vi "Update New Plugin by Reference.vi"(8 "error in (no error)":errorcluster, 10 "Plugin Types Tree":refnum<vi>, 11 "New Plugin Control":refnum<vi>) -> (0 "error out":errorcluster)   [LabVIEW 2021, in "CIF_Manager_UI.lvclass"]
uses:
  CIF_Manager_UI.lvclass
  Typedef/New Plugin.ctl
  CIF_Manager_UI.lvclass/CIF_Manager_UI.ctl
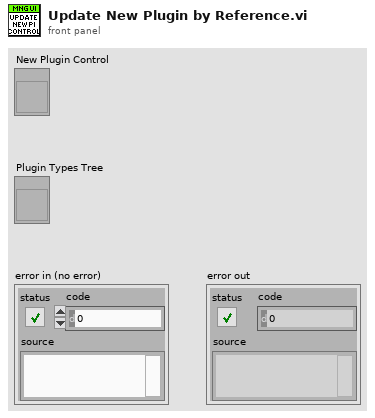
[diagram p1: front panel]
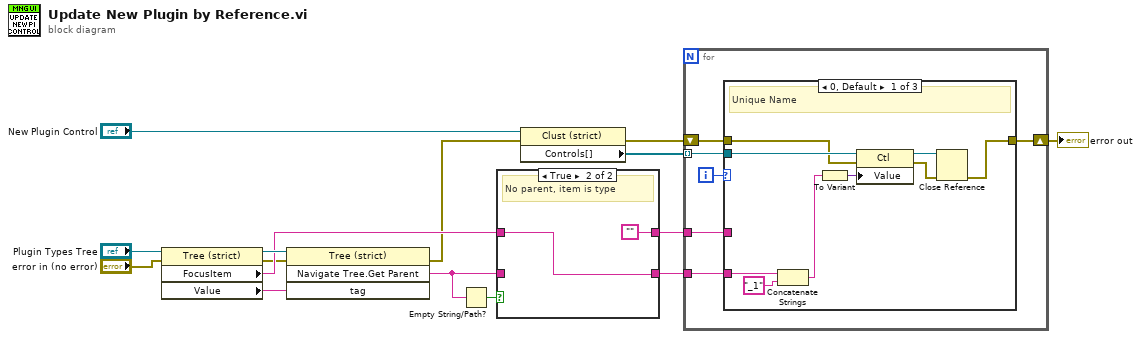
[diagram p0: block diagram]
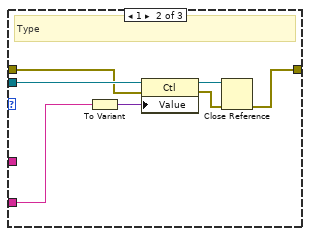
[diagram p3: hidden frame]
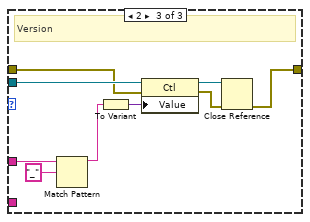
[diagram p4: hidden frame]
diagram:
  n1 = property class="Tree (strict)"(reference="Plugin Types Tree", error in="error in (no error)") -> (error out=w7:errorcluster, "FocusItem"=w8:string, "Value"=w13:string)  [unwired: 1 out]
  n2 = invoke class="Tree (strict)" method="Navigate Tree.Get Parent"(reference="Plugin Types Tree", error in=w7, "tag"=w13) -> (error out=w6:errorcluster, "Navigate Tree:Get Parent"=w9:string)  [unwired: 1 in, 2 out]
  n3 = Empty String/Path?(string/path=w9) -> (empty?=w10:bool)
  n4 = case shown="True" w10 {
    tunnel: w9 -> [w15 _]
    tunnel: w8 -> [w16 w18]
    tunnel: [w16 ""] -> w4
    tunnel: [w15 w18] -> w5
    frame False {
      # "Parent is type, item is version"
    }
    frame True {
      # "No parent, item is type"
    }
  }
  n5 = property class="Clust (strict)"(reference="New Plugin Control", error in=w6) -> (error out=w3:errorcluster, "Controls[]"=w14:refnum<vi>[])  [unwired: 1 out]
  n6 = for {
    tunnel: w14 -> [w23] mode=indexing
    tunnel: w5 -> [w22]
    tunnel: w4 -> [w21]
    shift-right: [w19] -> w1
    shift-left: w3 -> [w20]
    i -> [w24]
    n7 = case shown="0, Default" w24 {
      tunnel: w23 -> [w32 w40 w49]
      tunnel: w22 -> [w28 w38 _]
      tunnel: w21 -> [_ _ w43]
      tunnel: w20 -> [w30 w37 w47]
      tunnel: [w33 w34 w44] -> w19
      frame 0, Default {
        # "Unique Name"
        n8 = Concatenate Strings(w28, "_1" ("string")) -> (w26:string)
        n9 = To Variant(anything=w26) -> (Variant=w25:variant)
        n10 = property class="Ctl"(reference=w32, error in=w30, "Value"=w25) -> (reference out=w31:refnum<vi>, error out=w29:errorcluster)
        n11 = Close Reference(reference=w31, error in (no error)=w29) -> (error out=w33:errorcluster)
      }
      frame 1 {
        # "Type"
        n12 = To Variant(anything=w38) -> (Variant=w39:variant)
        n13 = property class="Ctl"(reference=w40, error in=w37, "Value"=w39) -> (reference out=w36:refnum<vi>, error out=w35:errorcluster)
        n14 = Close Reference(reference=w36, error in (no error)=w35) -> (error out=w34:errorcluster)
      }
      frame 2 {
        # "Version"
        n15 = Match Pattern(string=w43, regular expression="_") -> (before substring=w41:string)  [unwired: 1 in, 3 out]
        n16 = To Variant(anything=w41) -> (Variant=w48:variant)
        n17 = property class="Ctl"(reference=w49, error in=w47, "Value"=w48) -> (reference out=w46:refnum<vi>, error out=w45:errorcluster)
        n18 = Close Reference(reference=w46, error in (no error)=w45) -> (error out=w44:errorcluster)
      }
    }
  }
  "error out" <- w1
